vi "Stop Core.vi"(10 "final error code":i32, 11 "Actor_log in":refnum<class "Actor_log.lvclass">) -> (3 "Actor_log out":refnum<class "Actor_log.lvclass">)   [LabVIEW 2020, in "Actor_log.lvlib" / "Actor_log.lvclass"]
doc: "(<B>Filename</B>: Actor Framework.lvlib:Actor.lvclass:Stop Core.vi)\n\nDefines what the actor does before it stops. Use the <B>final error code</B> input to determine whether the actor shut down in response to an error.\n\nBy default, this method passes the Stop message along to all auto-stop nested actors. A descendant class may override this method to define additional behavior, such as shutting down any processes the actor initiated in its override of the Actor Core method."
uses:
  Actor_log.lvclass
  Actor_log.lvclass/Actor_log.ctl
  <vilib>/ActorFramework/Actor/Actor.lvclass
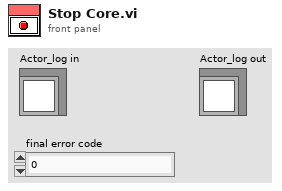
[diagram p1: front panel]
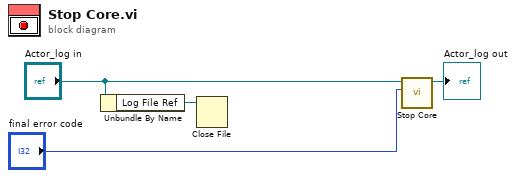
[diagram p0: block diagram]
diagram:
  n1 = Unbundle By Name("Actor_log in") -> ("Log File Ref"=w1:refnum<file>)
  n2 = Close File(refnum=w1) -> ()  [unwired: 1 in, 2 out]
  n3 = call-parent "Stop Core.vi"("final error code"="final error code", "Actor in"="Actor_log in") -> ("Actor out"=→"Actor_log out":refnum<class "Actor_log.lvclass">)  [unwired: 9 in]
